vi "Plot Time Range.vi"(8 "End":dbl format="%<%H:%M:%S%1u>T", 9 "Start":dbl format="%<%H:%M:%S%1u>T", 11 "Plot Data":cluster{"X":dbl[], "Y":dbl[]}) -> (0 "Actual End":dbl format="%<%H:%M:%S%1u>T", 1 "Actual Start":dbl format="%<%H:%M:%S%1u>T", 2 "X":dbl[](array[numeric]), 3 "Y":dbl[](array[numeric]))   [LabVIEW 2020, in "VolatusGUIElements.lvlib"]
uses:
  VolatusGUIElements.lvlib
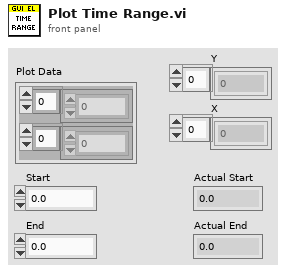
[diagram p1: front panel]
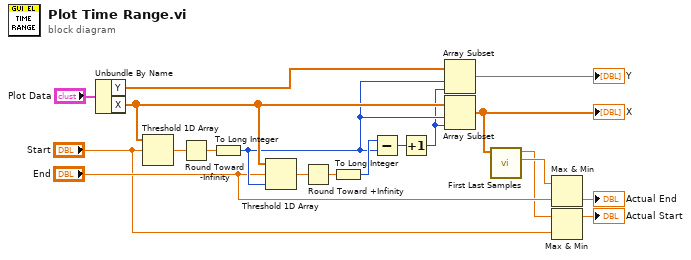
[diagram p0: block diagram]
diagram:
  n1 = Unbundle By Name("Plot Data") -> ("Y"=w12:dbl[], "X"=w11:dbl[])
  n2 = Threshold 1D Array(2:"Start", 3:w11) -> (0:w18:dbl)  [unwired: 1 in]
  n3 = Round Toward -Infinity(1:w18) -> (0:w17:dbl)
  n4 = To Long Integer(number=w17) -> (32bit integer=w10:i32)
  n5 = Threshold 1D Array(1:w10, 2:"End", 3:w11) -> (0:w16:dbl)
  n6 = Round Toward +Infinity(x=w16) -> (ceil(x): smallest int >= x=w15:dbl)
  n7 = To Long Integer(number=w15) -> (32bit integer=w14:i32)
  n8 = Subtract(x=w14, y=w10) -> (x-y=w13:i32)
  n9 = Increment(x=w13) -> (x+1=w9:i32)
  n10 = Array Subset(array=w12, index=w10, length=w9) -> (→"Y":dbl[])
  n11 = Array Subset(array=w11, index=w10, length=w9) -> (w7:dbl[])
  "X" <- w7
  n12 = call "First Last Samples.vi"("Data"=w7) -> ("Last"=w6:dbl, "First"=w3:dbl)  [unwired: 9 in]
  n13 = Max & Min(x=w6, y="End") -> (min(x,y)=→"Actual End":dbl)  [unwired: 1 out]
  n14 = Max & Min(x=w3, y="Start") -> (max(x,y)=→"Actual Start":dbl)  [unwired: 1 out]
